vi "drawLineToCenter.vi"(5 "ycenter":dbl, 7 "xcenter":dbl, 9 "yend":u32, 10 "ystart":dbl, 11 "xstart":dbl) -> (3 "xend":i32)   [LabVIEW 2020]
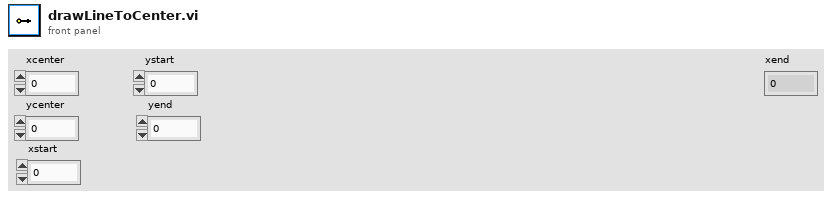
[diagram p1: front panel]
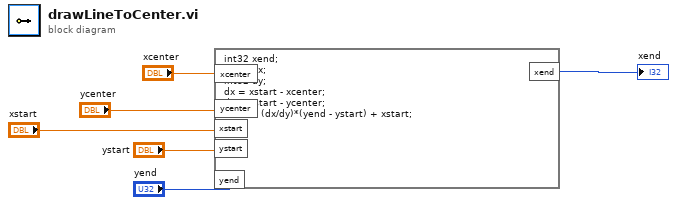
[diagram p0: block diagram]
diagram:
  n1 = formula code="int32 xend;\nint32 dx;\nint32 dy;\ndx = xstart - xcenter;\ndy = ystart - ycenter;\nxend = (dx/dy)*(yend - ystart) + xstart;"("ycenter"="ycenter", "xstart"="xstart", "ystart"="ystart", "xcenter"="xcenter", "yend"="yend") -> ("xend"=→"xend":i32)
